vi "BlinkCurrentProcess.vi"(8 "error in (no error)":errorcluster, 10 "index":i32, 11 "Status Control":refnum<vi>) -> (0 "error out":errorcluster)   [LabVIEW 2019]
doc: "Make the current process blink"
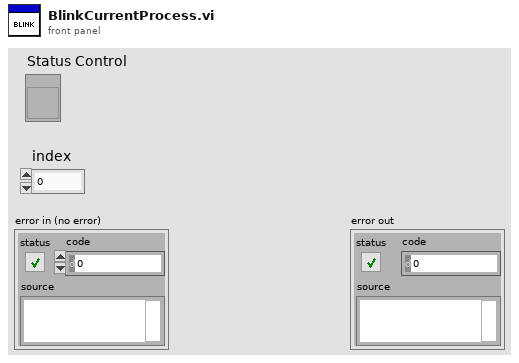
[diagram p1: front panel]
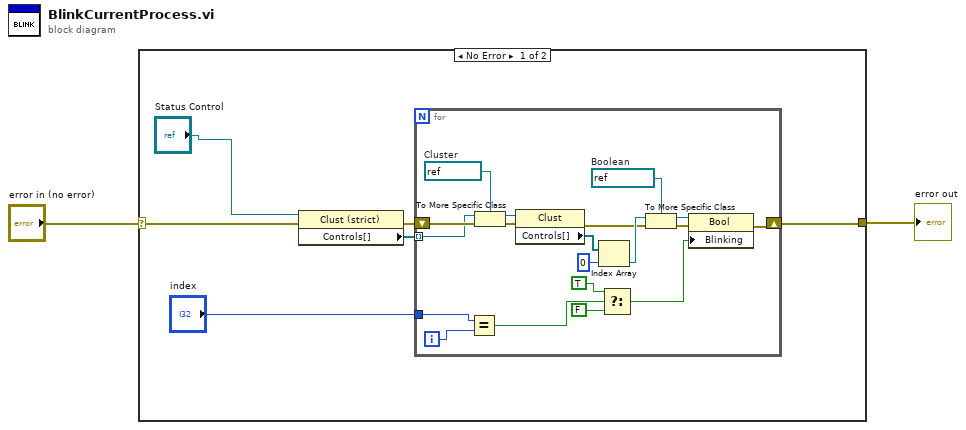
[diagram p0: block diagram]
diagram:
  n1 = case shown="No Error" "error in (no error)" {
    selector: "error in (no error)" -> [w6 w28]
    tunnel: [w4 w28] -> w1
    frame No Error {
      n2 = property class="Clust (strict)"(reference="Status Control", error in=w6) -> (error out=w7:errorcluster, "Controls[]"=w8:refnum<vi>[])  [unwired: 1 out]
      n3 = for {
        shift-right: [w20] -> w4
        shift-left: w7 -> [w16]
        tunnel: w8 -> [w15] mode=indexing
        tunnel: "index" -> [w14]
        i -> [w9]
        w19 = refnum<vi> refnum  # Cluster
        w25 = refnum<vi> refnum  # Boolean
        n4 = Equal?(x=w14, y=w9) -> (x = y?=w13:bool)
        n5 = To More Specific Class(target class=w19, reference=w15, error in=w16) -> (specific class reference=w18:refnum<vi>, error out=w17:errorcluster)
        n6 = property class="Clust"(reference=w18, error in=w17) -> (error out=w23:errorcluster, "Controls[]"=w26:refnum<vi>[])  [unwired: 1 out]
        n7 = Index Array(array=w26, index=0) -> (element=w24:refnum<vi>)
        n8 = Select(t=TRUE ("Blinking"), s=w13, f=FALSE) -> (s? t:f=w11:bool)
        n9 = To More Specific Class(target class=w25, reference=w24, error in=w23) -> (specific class reference=w22:refnum<vi>, error out=w21:errorcluster)
        n10 = property class="Bool"(reference=w22, error in=w21, "Blinking"=w11) -> (error out=w20:errorcluster)  [unwired: 1 out]
      }
    }
    frame Error {
    }
  }
  "error out" <- w1
